vi "SaveData.vi"(0 "object in":refnum<class "AFG3022B_OJ.lvclass">, 2 "tdms file":refnum<k34>, 5 "error in (no error)":errorcluster) -> (14 "object out":refnum<class "AFG3022B_OJ.lvclass">, 19 "error out":errorcluster)   [LabVIEW 2023, in "AFG3022B_OJ.lvclass"]
uses:
  AFG3022B_OJ.lvclass
  AFG3022B_OJ.lvclass/AFG3022B_OJ.ctl
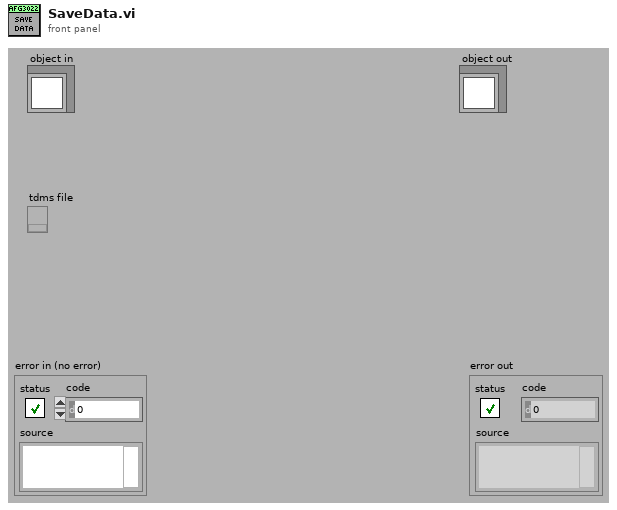
[diagram p1: front panel]
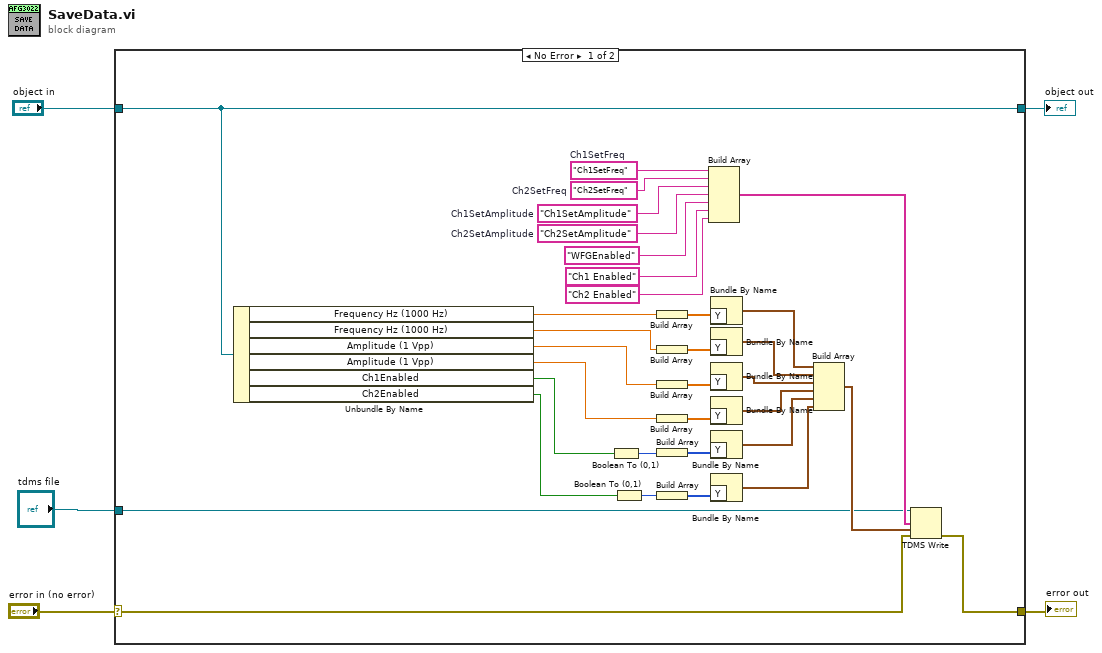
[diagram p0: block diagram]
diagram:
  n1 = case shown="No Error" "error in (no error)" {
    selector: "error in (no error)" -> [w8 w40]
    tunnel: [w7 w40] -> w4
    tunnel: [w38 w39] -> w2
    tunnel: "object in" -> [w38 w39]
    tunnel: "tdms file" -> [w6 _]
    frame No Error {
      w31 = "Ch2SetAmplitude"  # Ch2SetAmplitude
      w33 = "Ch2SetFreq"  # Ch2SetFreq
      w32 = "Ch1SetAmplitude"  # Ch1SetAmplitude
      w34 = "Ch1SetFreq"  # Ch1SetFreq
      n2 = Unbundle By Name(w38) -> ("Frequency Hz (1000 Hz)"=w18:dbl, "Frequency Hz (1000 Hz)"=w16:dbl, "Amplitude (1 Vpp)"=w15:dbl, "Amplitude (1 Vpp)"=w14:dbl, "Ch1Enabled"=w11:bool, "Ch2Enabled"=w9:bool)
      n3 = Boolean To (0,1)(Boolean=w11) -> (0, 1=w10:i16)
      n4 = Boolean To (0,1)(Boolean=w9) -> (0, 1=w20:i16)
      n5 = Build Array(w18) -> (w17:dbl[])
      n6 = Build Array(w16) -> (w37:dbl[])
      n7 = Build Array(w15) -> (w36:dbl[])
      n8 = Build Array(w14) -> (w35:dbl[])
      n9 = Build Array(w10) -> (w27:i16[])
      n10 = Build Array(w20) -> (w19:i16[])
      n11 = Build Array(w34, w33, w32, w31, "WFGEnabled", "Ch1 Enabled", "Ch2 Enabled") -> (w24:string[])
      n12 = Bundle By Name("Y"=w17) -> (w30:waveform(dbl))  [unwired: 1 in]
      n13 = Bundle By Name("Y"=w37) -> (w29:waveform(dbl))  [unwired: 1 in]
      n14 = Bundle By Name("Y"=w36) -> (w28:waveform(dbl))  [unwired: 1 in]
      n15 = Bundle By Name("Y"=w35) -> (w26:waveform(dbl))  [unwired: 1 in]
      n16 = Bundle By Name("Y"=w27) -> (w25:waveform(i16))  [unwired: 1 in]
      n17 = Bundle By Name("Y"=w19) -> (w21:waveform(i16))  [unwired: 1 in]
      n18 = Build Array(w30, w29, w28, w26, w25, w21) -> (w23:waveform(dbl)[])
      n19 = TDMS Write(0:w6, 7:w24, 9:w23, 11:w8) -> (15:w7:errorcluster)  [unwired: 2 in, 3 out]
    }
    frame Error {
    }
  }
  "error out" <- w4
  "object out" <- w2
